vi "Save States.vi"(8 "Error In":errorcluster, 9 "States Variant":variant, 10 "UIM Tag":refnum<k20>, 11 "XML Refnum":refnum<k20>) -> (0 "XML Error Out":errorcluster, 2 "UIM Tag Out":refnum<k20>, 3 "XML Refnum Out":refnum<k20>)   [LabVIEW 2015, in "UIM.lvclass"]
uses:
  UIM.lvclass
  UIP/UIP.lvclass
  <vilib>/xml/Close Reference(Node).vi
  <vilib>/xml/NI_XML.lvlib
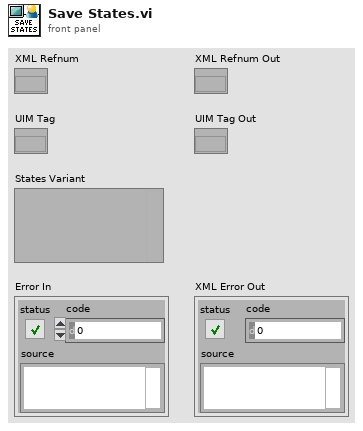
[diagram p1: front panel]
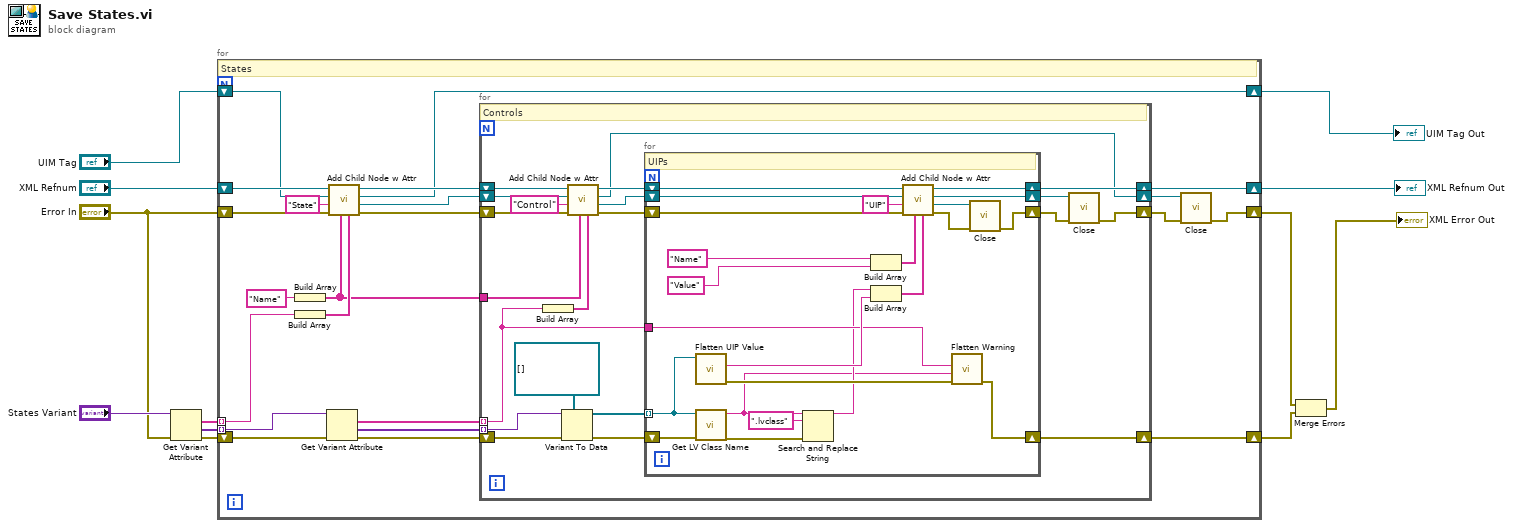
[diagram p0: block diagram]
diagram:
  n1 = Get Variant Attribute(Variant="States Variant", error in="Error In") -> (names=w12:string[], values=w11:variant[], error out=w10:errorcluster)  [unwired: 2 in, 1 out]
  n2 = for {
    tunnel: w12 -> [w32] mode=indexing
    tunnel: w11 -> [w16] mode=indexing
    shift-right: [w23] -> w7
    shift-left: w10 -> [w17]
    shift-right: [w18] -> w1
    shift-left: "Error In" -> [w29]
    shift-right: [w24] -> w8
    shift-left: "XML Refnum" -> [w34]
    shift-right: [w19] -> w2
    shift-left: "UIM Tag" -> [w31]
    # "States"
    n3 = Build Array("Name" ("Name")) -> (w25:string[])
    n4 = Build Array(w32) -> (w28:string[])
    n5 = Get Variant Attribute(Variant=w16, error in=w17) -> (names=w15:string[], values=w14:variant[], error out=w13:errorcluster)  [unwired: 2 in, 1 out]
    n6 = call "Add Child Node w Attr.vi"("Values"=w28, "Names"=w25, "Error In"=w29, "Tag Name"="State", "Parent Node"=w31, "DOM In"=w34) -> ("Error Out"=w26:errorcluster, "Child Node"=w22:refnum<k20>, "Parent Node"=w19:refnum<k20>, "DOM Out"=w27:refnum<k20>)  [unwired: 2 in]
    n7 = for {
      tunnel: w14 -> [w54] mode=indexing
      tunnel: w15 -> [w35] mode=indexing
      shift-right: [w42] -> w23
      shift-left: w13 -> [w53]
      tunnel: w25 -> [w47]
      shift-right: [w37] -> w20
      shift-left: w26 -> [w49]
      shift-right: [w43] -> w24
      shift-left: w27 -> [w51]
      shift-right: [w38] -> w21
      shift-left: w22 -> [w50]
      # "Controls"
      n8 = Build Array(w35) -> (w46:string[])
      n9 = Variant To Data(error in=w53, type=refnum<class "UIP.lvclass">[] [] ("UIP Defs"), Variant=w54) -> (data=w52:refnum<class "UIP.lvclass">[], error out=w36:errorcluster)
      n10 = call "Add Child Node w Attr.vi"("Values"=w46, "Names"=w47, "Error In"=w49, "Tag Name"="Control", "Parent Node"=w50, "DOM In"=w51) -> ("Error Out"=w44:errorcluster, "Child Node"=w41:refnum<k20>, "Parent Node"=w38:refnum<k20>, "DOM Out"=w45:refnum<k20>)  [unwired: 2 in]
      n11 = for {
        tunnel: w52 -> [w78] mode=indexing
        shift-right: [w68] -> w40
        shift-left: w44 -> [w76]
        shift-right: [w67] -> w43
        shift-left: w45 -> [w77]
        shift-right: [w60] -> w42
        shift-left: w36 -> [w63]
        shift-right: [w65] -> w39
        shift-left: w41 -> [w66]
        tunnel: w35 -> [w61]
        # "UIPs"
        n12 = call-dynamic "Flatten UIP Value.vi"("UIP In"=w78) -> ("Error Out"=w62:errorcluster, "String Value"=w71:string)  [unwired: 8 in, 1 out]
        n13 = call <vilib>:"Get LV Class Name.vi"("error in (no error)"=w63, "object"=w78) -> ("error out"=w57:errorcluster, "class name"=w56:string)  [unwired: 8 in]
        n14 = Search and Replace String(input string=w56, search string=".lvclass", error in=w57) -> (result string=w59:string)  [unwired: 5 in, 3 out]
        n15 = Build Array("Name" ("Name"), "Value" ("Name")) -> (w72:string[])
        n16 = Build Array(w59, w71) -> (w70:string[])
        n17 = call "Add Child Node w Attr.vi"("Values"=w70, "Names"=w72, "Error In"=w76, "Tag Name"="UIP", "Parent Node"=w66, "DOM In"=w77) -> ("Error Out"=w69:errorcluster, "Child Node"=w64:refnum<k20>, "Parent Node"=w65:refnum<k20>, "DOM Out"=w67:refnum<k20>)  [unwired: 2 in]
        n18 = call "Flatten Warning.vi"("Error In"=w62, "UIP Name"=w56, "Label.Text"=w61) -> ("Error Out"=w60:errorcluster)  [unwired: 8 in]
        n19 = call-poly <vilib>:"Close.vi"("error in (no error)"=w69, "node"=w64) -> ("error out"=w68:errorcluster)  [unwired: 7 in]
      }
      n20 = call-poly <vilib>:"Close.vi"("error in (no error)"=w40, "node"=w39) -> ("error out"=w37:errorcluster)  [unwired: 7 in]
    }
    n21 = call-poly <vilib>:"Close.vi"("error in (no error)"=w20, "node"=w21) -> ("error out"=w18:errorcluster)  [unwired: 7 in]
  }
  "XML Refnum Out" <- w8
  "UIM Tag Out" <- w2
  n22 = Merge Errors(w1, w7) -> (→"XML Error Out":errorcluster)
